vi "Test Audio Streamer.vi"() -> ()   [LabVIEW 2020]
uses:
  <vilib>/Analysis/NI_AALBase.lvlib
panel:
  out "streamer is open":bool
  out "Error message":string
  out "Status":string
  in  "Stop":bool
  in  "Start":bool
  in  "Trigger":bool
  out "Waveform Graph":dbl[][](graph)
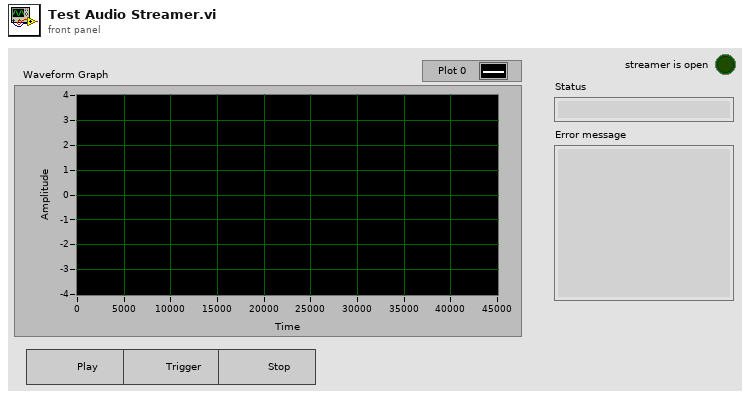
[diagram p1: front panel]
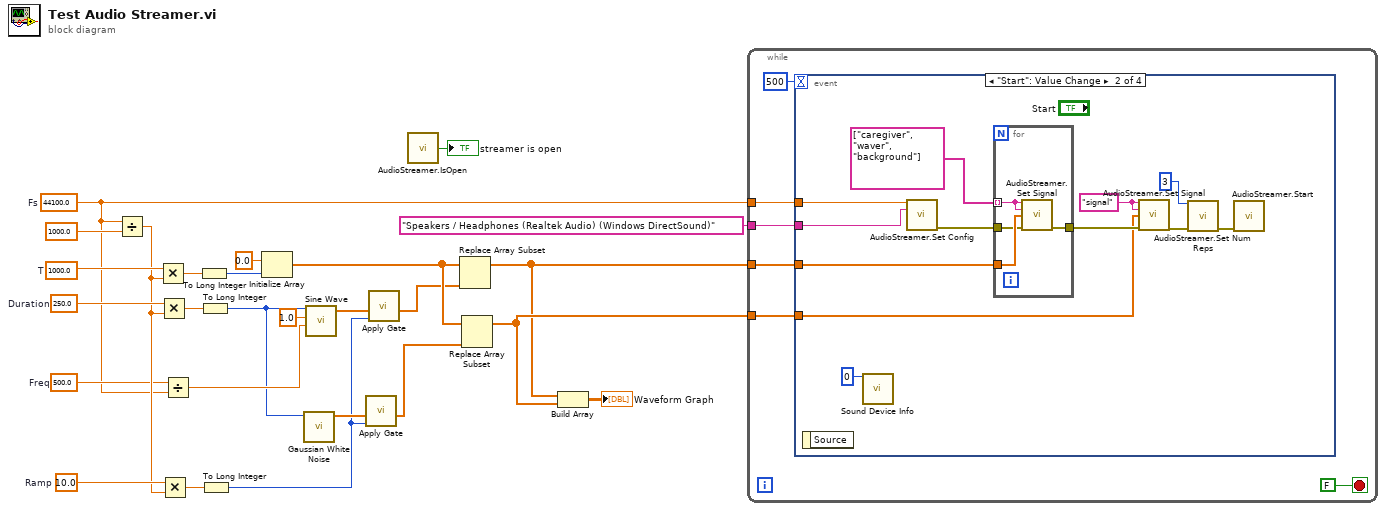
[diagram p0: block diagram]
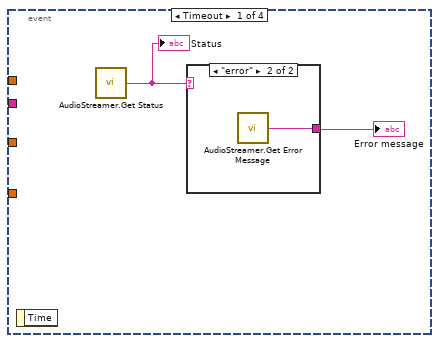
[diagram p2: hidden frame]
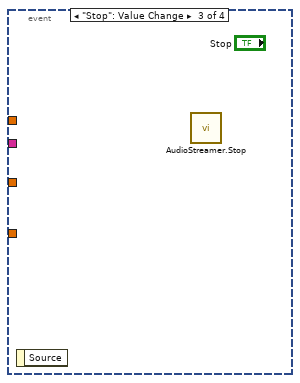
[diagram p4: hidden frame]
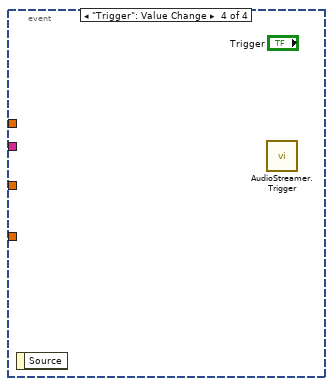
[diagram p5: hidden frame]
diagram:
  w15 = 500.0  # Freq
  w20 = 10.0  # Ramp
  w22 = 250.0  # Duration
  w25 = 1000.0  # T
  w6 = 44100.0  # Fs
  n1 = Divide(x=w6, y=1000.0) -> (x/y=w19:dbl)
  n2 = Multiply(x=w25, y=w19) -> (x*y=w24:dbl)
  n3 = Multiply(x=w22, y=w19) -> (x*y=w23:dbl)
  n4 = Multiply(x=w20, y=w19) -> (x*y=w21:dbl)
  n5 = Divide(x=w15, y=w6) -> (x/y=w14:dbl)
  n6 = To Long Integer(number=w24) -> (32bit integer=w18:i32)
  n7 = To Long Integer(number=w23) -> (32bit integer=w13:i32)
  n8 = To Long Integer(number=w21) -> (32bit integer=w9:i32)
  n9 = Initialize Array(0.0 ("element"), w18) -> (w12:dbl[])
  n10 = call <vilib>:"Gaussian White Noise.vi"("samples"=w13) -> ("Gaussian noise pattern"=w10:dbl[])  [unwired: 9 in, 1 out]
  n11 = call <vilib>:"Sine Wave.vi"("samples"=w13, "amplitude"=1.0, "frequency"=w14) -> ("sine wave"=w11:dbl[])  [unwired: 2 in, 2 out]
  n12 = call "Apply Gate.vi"("nramp"=w9, "Waveform in"=w10) -> ("Gated waveform"=w3:dbl[])  [unwired: 9 in]
  n13 = call "Apply Gate.vi"("nramp"=w9, "Waveform in"=w11) -> ("Gated waveform"=w4:dbl[])  [unwired: 9 in]
  n14 = call "AudioStreamer.IsOpen.vi"() -> ("success"=→"streamer is open":bool)  [unwired: 1 in]
  n15 = Replace Array Subset(array=w12, new element=w4) -> (w5:dbl[])  [unwired: 1 in]
  n16 = Replace Array Subset(array=w12, new element=w3) -> (w7:dbl[])  [unwired: 1 in]
  n17 = Build Array(w5, w7) -> (→"Waveform Graph":dbl[][])
  n18 = while {
    tunnel: w5 -> [w31]
    tunnel: w7 -> [w30]
    tunnel: w6 -> [w28]
    tunnel: "Speakers / Headphones (Realtek Audio) (Windows DirectSound)" -> [w27]
    stop <- FALSE stop-if-true
    n19 = event shown="[1] \"Start\": Value Change" {
      selector: _ -> [_ _ _ _]
      dyn-events: _ -> [_ _ _ _]
      timeout: 500 -> [_ _ _ _]
      tunnel: w31 -> [_ w44 _ _]
      tunnel: w30 -> [_ w41 _ _]
      tunnel: w28 -> [_ w47 _ _]
      tunnel: w27 -> [_ w39 _ _]
      event Timeout {
        n20 = event-data() -> ()  [unwired: 1 in, 1 out]
        n21 = call "AudioStreamer.Get Status.vi"() -> ("status"=w34:string)  [unwired: 1 in]
        "Status" <- w34
        n22 = case shown="\"error\"" w34 {
          tunnel: [_ w35] -> w33
          frame "", Default {
          }
          frame "error" {
            n23 = call "AudioStreamer.Get Error Message.vi"() -> ("message"=w35:string)  [unwired: 1 in]
          }
        }
        "Error message" <- w33
      }
      event "Start": Value Change {
        w40 = "signal" ("destination")
        n24 = event-data() -> ()  [unwired: 1 in, 1 out]
        n25 = call <vilib>:"Sound Device Info.vi"("device"=u32 0) -> ()  [unwired: 12 in, 3 out]
        n26 = call "AudioStreamer.Set Config.vi"("Fs (Hz)"=w47, "device"=w39) -> ("error out"=w43:errorcluster)  [unwired: 13 in]
        n27 = for {
          tunnel: string[] ["caregiver", "waver", "background"] -> [w48] mode=indexing
          tunnel: w44 -> [w51]
          tunnel: w43 -> [w50]
          tunnel: [w49] -> w42
          n28 = call "AudioStreamer.Set Signal.vi"("destination"=w48, "name"=w48, "data"=w51, "error in (no error)"=w50) -> ("error out"=w49:errorcluster)  [unwired: 11 in]
        }
        n29 = call "AudioStreamer.Set Signal.vi"("destination"=w40, "name"=w40, "data"=w41, "error in (no error)"=w42) -> ("error out"=w38:errorcluster)  [unwired: 11 in]
        n30 = call "AudioStreamer.Set Num Reps.vi"("nreps"=3, "error in (no error)"=w38) -> ("error out"=w37:errorcluster)  [unwired: 13 in]
        n31 = call "AudioStreamer.Start.vi"("error in (no error)"=w37) -> ()  [unwired: 14 in, 1 out]
      }
      event "Stop": Value Change {
        n32 = event-data() -> ()  [unwired: 1 in, 1 out]
        n33 = call "AudioStreamer.Stop.vi"() -> ()  [unwired: 15 in, 1 out]
      }
      event "Trigger": Value Change {
        n34 = event-data() -> ()  [unwired: 1 in, 1 out]
        n35 = call "AudioStreamer.Trigger.vi"() -> ()  [unwired: 15 in, 1 out]
      }
    }
  }
